vi "SaveP1.vi"(11 "OSA Setting":T1) -> (1 "Power":dbl[](array[numeric]), 3 "Wavelength":dbl[](array[numeric]))   [LabVIEW 2020]
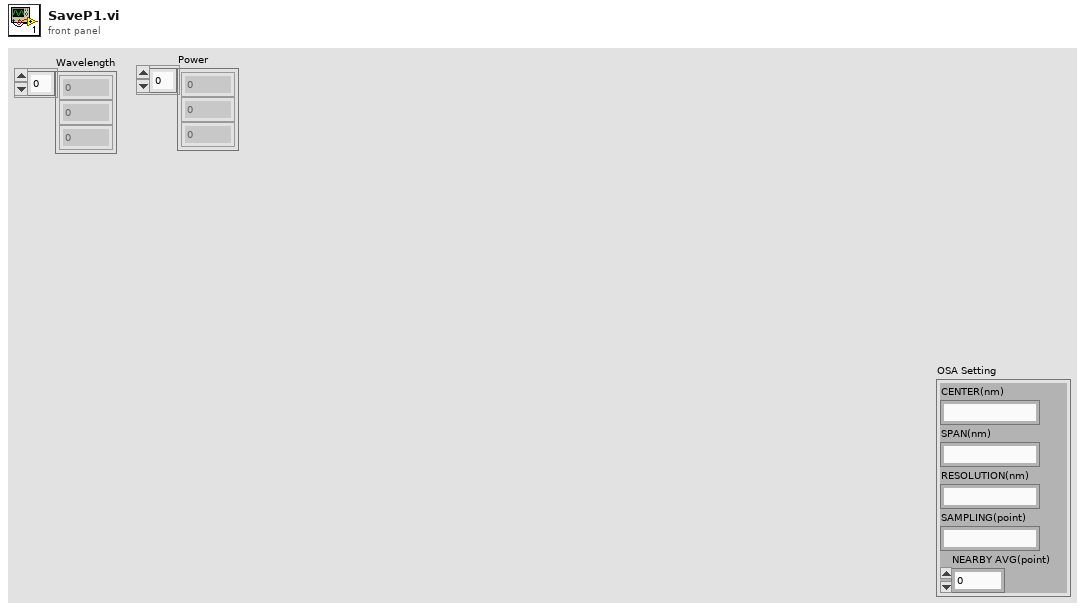
[diagram p1: front panel]
types:
  T1 = cluster{"CENTER(nm)":string, "SPAN(nm)":string, "RESOLUTION(nm)":string, "SAMPLING(point)":string, "NEARBY AVG(point)":i32}
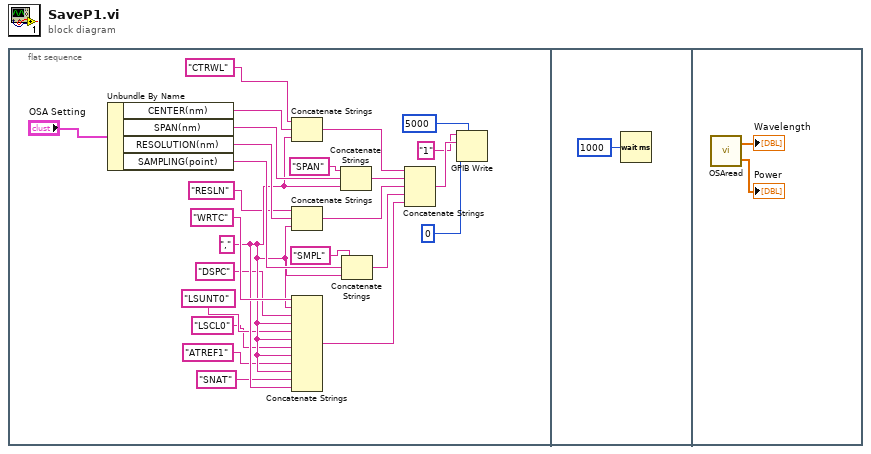
[diagram p0: block diagram]
diagram:
  n1 = flat-sequence {
    frame #0 {
      w13 = ","
      n2 = Unbundle By Name("OSA Setting") -> ("CENTER(nm)"=w15:string, "SPAN(nm)"=w16:string, "RESOLUTION(nm)"=w17:string, "SAMPLING(point)"=w18:string)
      n3 = Concatenate Strings("CTRWL", w15, w13) -> (w19:string)
      n4 = Concatenate Strings("RESLN", w17, w13) -> (w21:string)
      n5 = Concatenate Strings("WRTC", w13, "DSPC", w13, "LSUNT0", w13, "LSCL0", w13, "ATREF1", w13, "SNAT", w13) -> (w24:string)
      n6 = Concatenate Strings("SPAN", w16, w13) -> (w20:string)
      n7 = Concatenate Strings("SMPL", w18, w13) -> (w22:string)
      n8 = Concatenate Strings(w19, w20, w21, w22, w24) -> (w23:string)
      n9 = GPIB Write(0:"1" ("address string"), 1:w23, 2:i16 0 ("mode (0)"), 4:5000 ("timeout ms (488.2 global)")) -> ()  [unwired: 1 in, 2 out]
    }
    frame #1 {
      n10 = Wait (ms)(milliseconds to wait=u32 1000) -> ()  [unwired: 1 out]
    }
    frame #2 {
      n11 = call "OSAread.vi"() -> ("power"=→"Power":dbl[], "length"=→"Wavelength":dbl[])  [unwired: 2 out]
    }
  }
